vi "VstepGlobal.vi"() -> ()   [LabVIEW 2011]
panel:
  in  "V step [V]":dbl=0.001
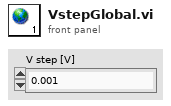
[diagram p1: front panel]
diagram:
